vi "test_ccd_roi.vi"(8 "error in":errorcluster, 11 "CCD in":refnum<class "CCD.lvclass">) -> (0 "error out":errorcluster, 3 "CCD out":refnum<class "CCD.lvclass">)   [LabVIEW 2023, in "horiba.test.lvlib"]
uses:
  horiba.test.lvlib
  Classes/CCD/CCD.lvclass
  C:/Projects/Horiba/horiba-labview-sdk/Source/Classes/GenericDevice/GenericDevice.lvclass
  <vilib>/addons/_JKI Toolkits/Caraya/classes/Assert/Assert Equal Value_Variant.vi
  <vilib>/addons/_JKI Toolkits/Caraya/classes/Test/Test.lvclass
  <vilib>/addons/_JKI Toolkits/Caraya/classes/Assert/Assert.lvclass
  <userlib>/_OpenG.lib/lvdata/lvdata.llb/openg_variant.lvlib
panel:
  # "Connector Pane"
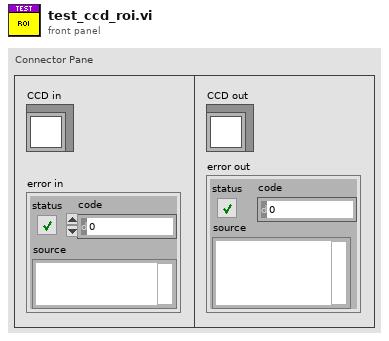
[diagram p1: front panel]
types:
  T1 = cluster{"ROI-index":i32, "xOrigin":i32, "yOrigin":i32, "xSize":i32, "ySize":i32, "xBin":i32, "yBin":i32}
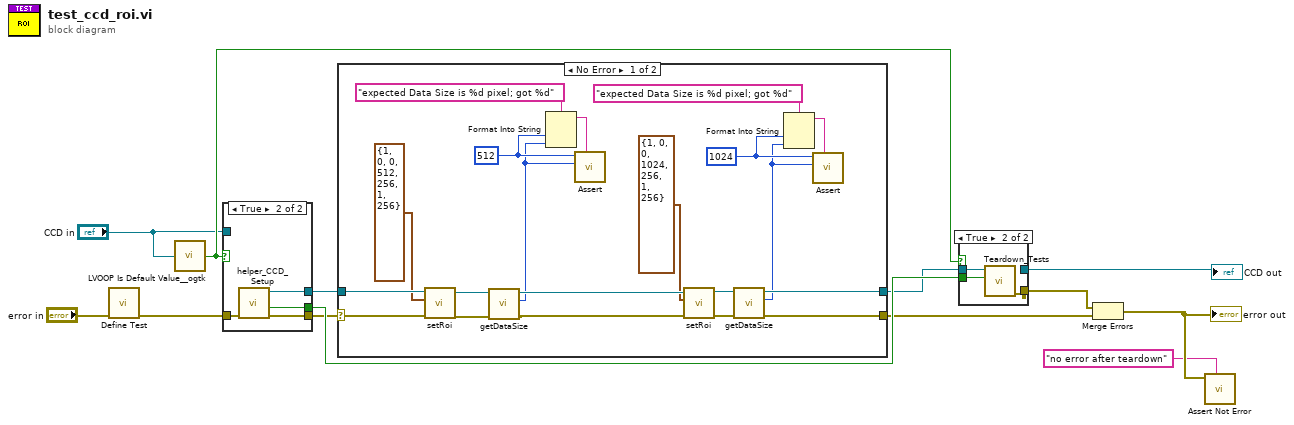
[diagram p0: block diagram]
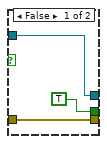
[diagram p2: hidden frame]
diagram:
  n1 = call <vilib>:"Define Test.vi"("error in (no error)"="error in") -> ("error out"=w8:errorcluster)  [unwired: 9 in, 1 out]
  n2 = call <userlib>:"LVOOP Is Default Value__ogtk.vi"("Object"="CCD in") -> ("Is Default Value?"=w9:bool)
  n3 = case shown="True" w9 {
    tunnel: w8 -> [w15 w20]
    tunnel: [w15 w19] -> w4
    tunnel: [w16 w18] -> w6
    tunnel: [TRUE ("Module Was Already Running?") w17] -> w10
    tunnel: "CCD in" -> [w16 _]
    frame False {
    }
    frame True {
      n4 = call "helper_CCD_Setup.vi"("error in"=w20) -> ("error out"=w19:errorcluster, "Module Was Already Running?"=w17:bool, "CCD out"=w18:refnum<class "CCD.lvclass">)  [unwired: 7 in, 1 out]
    }
  }
  n5 = case shown="No Error" w4 {
    selector: w4 -> [w39 w41]
    tunnel: [w24 w42] -> w5
    tunnel: w6 -> [w40 w42]
    tunnel: [w26 w41] -> w3
    frame No Error {
      w28 = 1024 ("size")
      w32 = 512 ("size")
      n6 = call "setRoi.vi"("error in (no error)"=w39, "roiConfig"=T1 {"ROI-index"=1, "xOrigin"=0, "yOrigin"=0, "xSize"=512, "ySize"=256, "xBin"=1, "yBin"=256}, "CCD in"=w40) -> ("error out"=w37:errorcluster, "CCD out"=w38:refnum<class "CCD.lvclass">)  [unwired: 5 in, 2 out]
      n7 = call "getDataSize.vi"("error in (no error)"=w37, "CCD in"=w38) -> ("error out"=w36:errorcluster, "size"=w31:i32, "CCD out"=w34:refnum<class "CCD.lvclass">)  [unwired: 7 in]
      n8 = Format Into String(format string="expected Data Size is %d pixel; got %d" ("Label"), w32, w31) -> (resulting string=w30:string)  [unwired: 2 in, 1 out]
      n9 = call-poly <vilib>:"Assert.vi"("Label"=w30, "Y"=w31, "X"=w32) -> ()  [unwired: 7 in, 2 out]
      n10 = call "setRoi.vi"("error in (no error)"=w36, "roiConfig"=T1 {"ROI-index"=1, "xOrigin"=0, "yOrigin"=0, "xSize"=1024, "ySize"=256, "xBin"=1, "yBin"=256}, "CCD in"=w34) -> ("error out"=w35:errorcluster, "CCD out"=w25:refnum<class "CCD.lvclass">)  [unwired: 5 in, 2 out]
      n11 = call "getDataSize.vi"("error in (no error)"=w35, "CCD in"=w25) -> ("error out"=w26:errorcluster, "size"=w23:i32, "CCD out"=w24:refnum<class "CCD.lvclass">)  [unwired: 7 in]
      n12 = Format Into String(format string="expected Data Size is %d pixel; got %d" ("Label"), w28, w23) -> (resulting string=w29:string)  [unwired: 2 in, 1 out]
      n13 = call-poly <vilib>:"Assert.vi"("Label"=w29, "Y"=w23, "X"=w28) -> ()  [unwired: 7 in, 2 out]
    }
    frame Error {
    }
  }
  n14 = case shown="True" w9 {
    tunnel: w5 -> [w43 w46]
    tunnel: [_ w45] -> w7
    tunnel: w10 -> [_ w44]
    tunnel: [w43 _] -> w1
    frame False {
    }
    frame True {
      n15 = call "Teardown_Tests.vi"("Module Was Already Running?"=w44, "horiba.lvlib:GenericDevice"=w46) -> ("error out"=w45:errorcluster)  [unwired: 8 in, 1 out]
    }
  }
  "CCD out" <- w1
  n16 = Merge Errors(w7, w3) -> (w12:errorcluster)
  "error out" <- w12
  n17 = call <vilib>:"Assert Not Error.vi"("Label"="no error after teardown", "Not Error?"=w12) -> ()  [unwired: 8 in, 2 out]
